vi "Th2829NX_PAGE_TSD2.vi"(8 "错误输入（无错误）":errorcluster, 11 "VISA资源名称":refnum<visa-resource-name>) -> (0 "error out":errorcluster, 3 "VISA资源名称输出":refnum<visa-resource-name>)   [LabVIEW 2018]
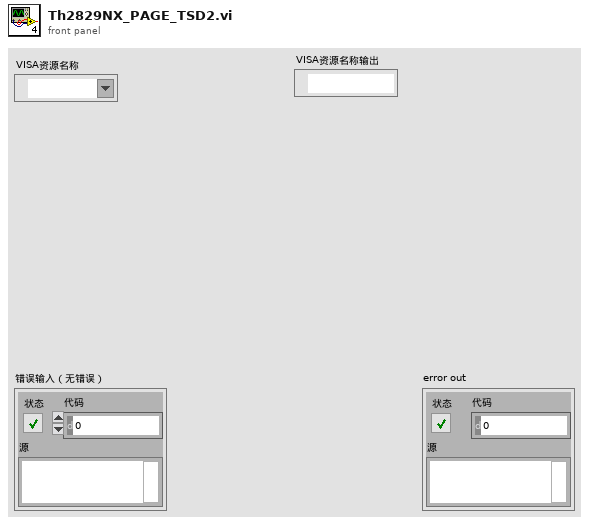
[diagram p1: front panel]
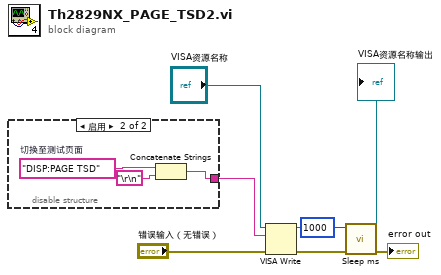
[diagram p0: block diagram]
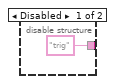
[diagram p2: hidden frame]
diagram:
  n1 = disable-structure shown="启用" {
    disable-tunnel: ["trig" ("write buffer") w9] -> w6
    frame Disabled {
    }
    frame Enabled {
      w10 = "DISP:PAGE TSD"  # 切换至测试页面
      n2 = Concatenate Strings(w10, "\r\n") -> (w9:string)
    }
  }
  n3 = VISA Write(VISA resource name="VISA资源名称", write buffer=w6, error in (no error)="错误输入（无错误）") -> (VISA resource name out=→"VISA资源名称输出":refnum<visa-resource-name>, error out=w2:errorcluster)  [unwired: 1 out]
  n4 = call "Sleep ms.vi"("error in (no error)"=w2, "等待时间（毫秒）"=u32 1000) -> ("error out"=→"error out":errorcluster)  [unwired: 9 in]
